vi "TypeToVariantForContextHelp.vi"(11 "Type":refnum<class "Type.lvclass">) -> (3 "Variant":variant)   [LabVIEW 2021]
uses:
  <vilib>/imath/engines/lvmath2/MathScriptCompiler/Type.llb/Type.lvclass
  <vilib>/imath/engines/lvmath2/MathScriptCompiler/Type/Matrix.llb/Matrix.lvclass
  C:/builds/2021/dev/dist/vi.lib/imath/engines/lvmath2/MathScriptCompiler/Type/NDArray.llb/NDArray.lvclass
  C:/builds/2021/dev/dist/vi.lib/imath/engines/lvmath2/MathScriptCompiler/Type.llb/Type.lvclass
  <vilib>/imath/engines/lvmath2/MathScriptCompiler/Type/BaseEltType.llb/BaseEltType.lvclass
  <vilib>/imath/engines/lvmath2/MathScriptCompiler/Type/PlugInEltType.llb/PlugInEltType.lvclass
  <vilib>/Utility/VariantDataType/MemoryInfo.ctl
  <vilib>/Utility/VariantDataType/MemoryType.ctl
  <vilib>/imath/engines/lvmath2/MathScriptCompiler/Type/NDArray.llb/NDArray.lvclass
  <vilib>/imath/engines/lvmath2/MathScriptCompiler/Type/StructEltType.llb/StructEltType.lvclass
  <vilib>/Utility/VariantDataType/VariantType.lvlib
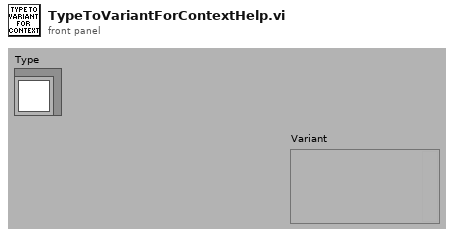
[diagram p1: front panel]
types:
  T1 = typedef "VariantType.lvlib/MemoryInfo.ctl" = cluster{"Type":T2, "Size":u32}
  T2 = typedef "VariantType.lvlib/MemoryType.ctl" = enum16{"Variable", "Fixed", "Bounded"}
  T3 = typedef "MathScriptTypes.lvlib/Matrix.lvclass/Shape.ctl" = enum16{"Scalar", "Row Vector", "Column Vector", "Matrix"}
  T4 = typedef "MathScriptTypes.lvlib/StructEltType.lvclass/StructField.ctl" = cluster{"Name":string, "Data Type":refnum<class "Type.lvclass">}
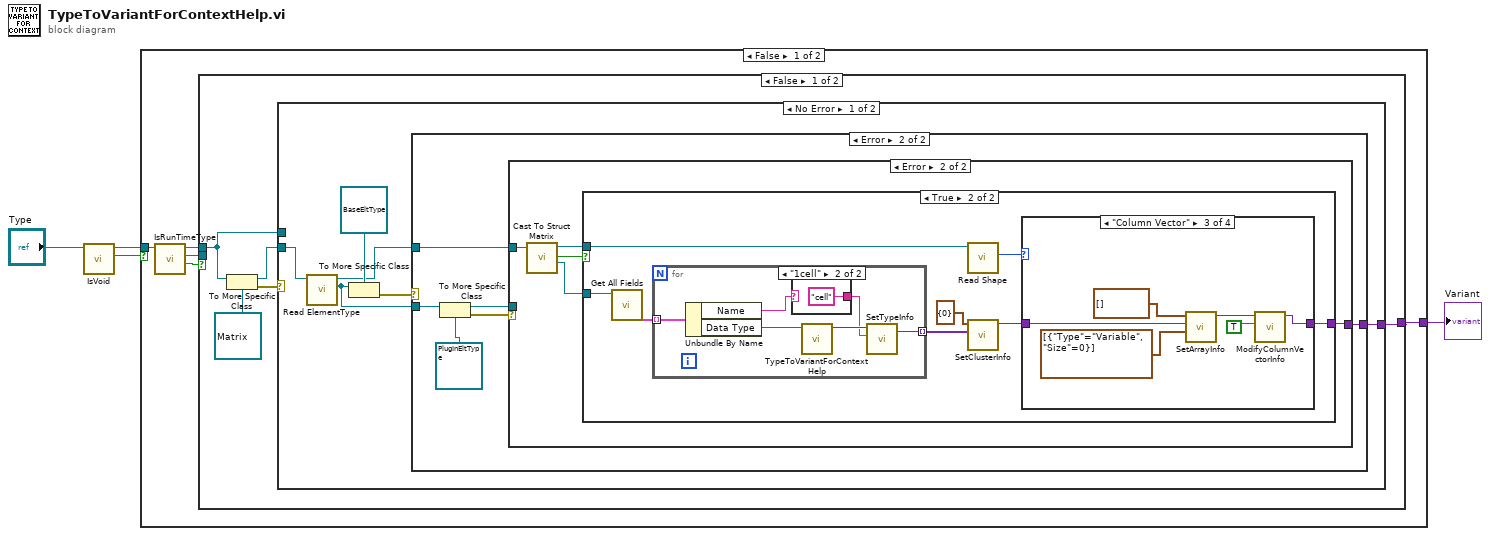
[diagram p0: block diagram]
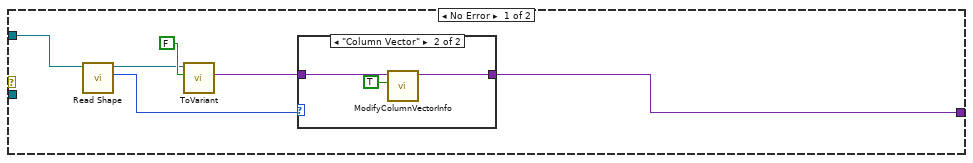
[diagram p2: hidden frame]
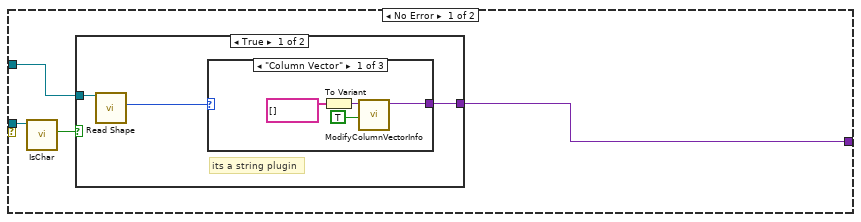
[diagram p4: hidden frame]
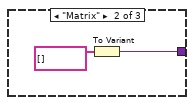
[diagram p5: hidden frame]
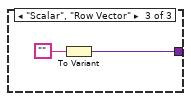
[diagram p6: hidden frame]
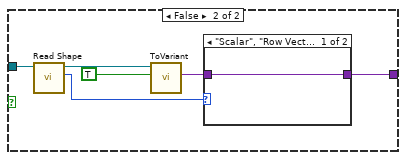
[diagram p7: hidden frame]
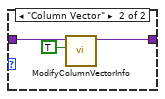
[diagram p8: hidden frame]
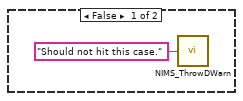
[diagram p9: hidden frame]
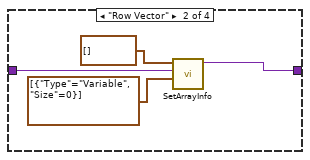
[diagram p11: hidden frame]
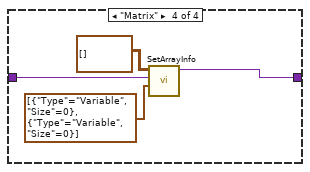
[diagram p12: hidden frame]
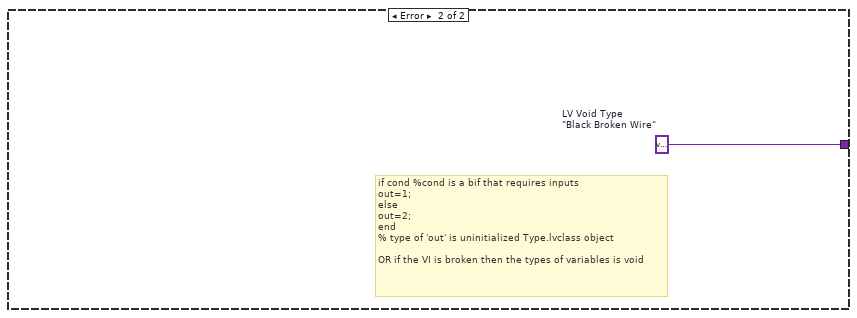
[diagram p14: hidden frame]
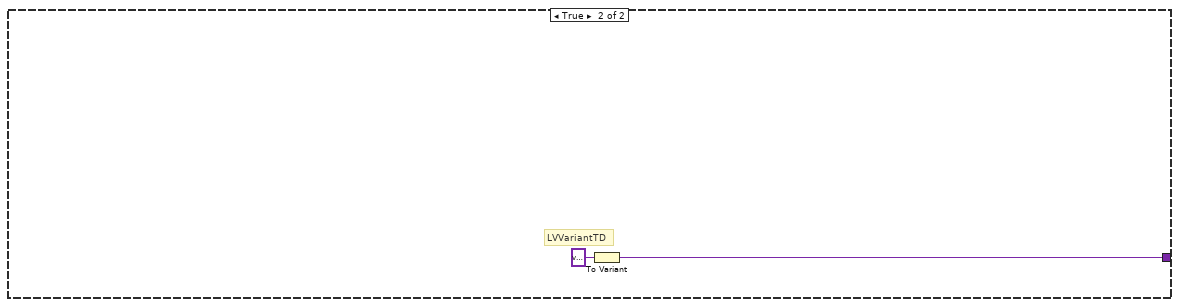
[diagram p15: hidden frame]
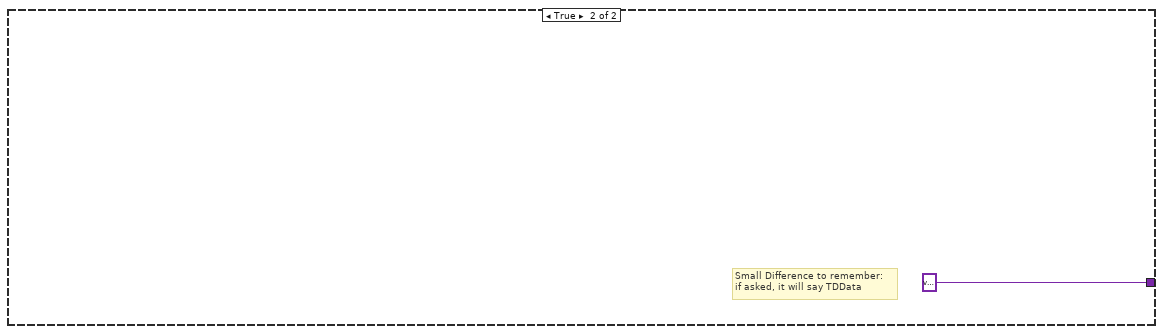
[diagram p16: hidden frame]
diagram:
  n1 = call-dynamic "IsVoid.vi"("Type in"="Type") -> ("IsVoid"=w1:bool, "Type out"=w2:refnum<class "Type.lvclass">)  [unwired: 9 in]
  n2 = case shown="False" w1 {
    tunnel: [w6 variant ("Variant")] -> w4
    tunnel: w2 -> [w5 _]
    frame False {
      n3 = call-dynamic "IsRunTimeType.vi"("Type"=w5) -> ("IsRunTimeType?"=w7:bool, "RunTimeType out"=w9:refnum<class "RuntimeType.lvclass">, "Type (dup)"=w8:refnum<class "Type.lvclass">)  [unwired: 8 out]
      n4 = case shown="False" w7 {
        tunnel: w9 -> [_ _]
        tunnel: w8 -> [w10 _]
        tunnel: [w11 w100] -> w6
        frame False {
          n5 = To More Specific Class(target class=refnum<class "Matrix.lvclass"> refnum ("Matrix out"), reference=w10) -> (specific class reference=w12:refnum<class "Matrix.lvclass">, error out=w13:errorcluster)  [unwired: 1 in]
          n6 = case shown="No Error" w13 {
            tunnel: w12 -> [w19 _]
            tunnel: [w15 w99] -> w11
            tunnel: w10 -> [_ _]
            frame No Error {
              n7 = call <vilib>:"Read ElementType.vi"("NDArray.lvclass in"=w19) -> ("ElementType"=w16:refnum<class "ElementType.lvclass">, "NDArray.lvclass out"=w17:refnum<class "Matrix.lvclass">)  [unwired: 9 out]
              n8 = To More Specific Class(target class=refnum<class "BaseEltType.lvclass"> refnum ("BaseEltType.lvclass in"), reference=w16) -> (error out=w18:errorcluster)  [unwired: 1 in, 1 out]
              n9 = case shown="Error" w18 {
                tunnel: w17 -> [w25 w32]
                tunnel: [w21 w31] -> w15
                tunnel: w16 -> [_ w35]
                frame No Error {
                  n10 = call <vilib>:"Read Shape.vi"("Matrix.lvclass in"=w25) -> ("Shape"=w23:T3, "Matrix.lvclass out"=w24:refnum<class "Matrix.lvclass">)  [unwired: 9 in]
                  n11 = call-dynamic "ToVariant.vi"("Set ColVector on TDR? (F)"=FALSE ("Ignore CondDefined?"), "Matrix in"=w24) -> ("Variant"=w22:variant)  [unwired: 2 in, 7 out]
                  n12 = case shown="\"Column Vector\"" w23 {
                    tunnel: w22 -> [w27 w28]
                    tunnel: [w27 w30] -> w21
                    frame "Scalar", "Row Vector", "Matrix" {
                    }
                    frame "Column Vector" {
                      n13 = call <vilib>:"ModifyColumnVectorInfo.vi"("isColumnVector"=TRUE, "Variant"=w28) -> ("Variant out"=w30:variant)  [unwired: 8 in, 1 out]
                    }
                  }
                }
                frame Error {
                  n14 = To More Specific Class(target class=refnum<class "PlugInEltType.lvclass"> refnum, reference=w35) -> (specific class reference=w33:refnum<class "PlugInEltType.lvclass">, error out=w34:errorcluster)  [unwired: 1 in]
                  n15 = case shown="Error" w34 {
                    tunnel: w33 -> [w38 _]
                    tunnel: w32 -> [w40 w66]
                    tunnel: [w39 w62] -> w31
                    frame No Error {
                      n16 = call-dynamic "IsChar.vi"("PlugInEltType in"=w38) -> ("Is Char?"=w37:bool)  [unwired: 9 in, 1 out]
                      n17 = case shown="True" w37 {
                        tunnel: w40 -> [w43 w57]
                        tunnel: [w41 w52] -> w39
                        frame True {
                          # "its a string plugin"
                          n18 = call <vilib>:"Read Shape.vi"("Matrix.lvclass in"=w43) -> ("Shape"=w42:T3)  [unwired: 9 in, 1 out]
                          n19 = case shown="\"Column Vector\"" w42 {
                            tunnel: [w47 w48 w50] -> w41
                            frame "Column Vector" {
                              n20 = To Variant(anything=string[] []) -> (Variant=w45:variant)
                              n21 = call <vilib>:"ModifyColumnVectorInfo.vi"("isColumnVector"=TRUE, "Variant"=w45) -> ("Variant out"=w47:variant)  [unwired: 8 in, 1 out]
                            }
                            frame "Matrix" {
                              n22 = To Variant(anything=string[] []) -> (Variant=w48:variant)
                            }
                            frame "Scalar", "Row Vector" {
                              n23 = To Variant(anything="") -> (Variant=w50:variant)
                            }
                          }
                        }
                        frame False {
                          n24 = call <vilib>:"Read Shape.vi"("Matrix.lvclass in"=w57) -> ("Shape"=w56:T3, "Matrix.lvclass out"=w55:refnum<class "Matrix.lvclass">)  [unwired: 9 in]
                          n25 = call-dynamic "ToVariant.vi"("Set ColVector on TDR? (F)"=TRUE ("Ignore CondDefined?"), "Matrix in"=w55) -> ("Variant"=w53:variant)  [unwired: 7 in, 2 out]
                          n26 = case shown="\"Scalar\", \"Row Vector\", \"Matrix\"" w56 {
                            tunnel: w53 -> [w58 w61]
                            tunnel: [w58 w60] -> w52
                            frame "Scalar", "Row Vector", "Matrix" {
                            }
                            frame "Column Vector" {
                              n27 = call <vilib>:"ModifyColumnVectorInfo.vi"("isColumnVector"=TRUE, "Variant"=w61) -> ("Variant out"=w60:variant)  [unwired: 8 in, 1 out]
                            }
                          }
                        }
                      }
                    }
                    frame Error {
                      n28 = call <vilib>:"Cast To Struct Matrix.vi"("Type in"=w66) -> ("IsStructMatrix?"=w65:bool, "StructEltType out"=w64:refnum<class "StructEltType.lvclass">, "Type (dup)"=w63:refnum<class "Matrix.lvclass">)  [unwired: 7 in, 1 out]
                      n29 = case shown="True" w65 {
                        tunnel: w64 -> [_ w75]
                        tunnel: w63 -> [_ w73]
                        tunnel: [_ w71] -> w62
                        frame False {
                          n30 = call <vilib>:"NIMS_ThrowDWarn.vi"("DWarn"="Should not hit this case.") -> ()  [unwired: 1 in]
                        }
                        frame True {
                          n31 = call <vilib>:"Get All Fields.vi"("StructEltType in"=w75) -> ("Fields"=w74:T4[])  [unwired: 8 in, 2 out]
                          n32 = for {
                            tunnel: w74 -> [w96] mode=indexing
                            tunnel: [w93] -> w69 mode=indexing
                            n33 = Unbundle By Name(w96) -> ("Name"=w92:string, "Data Type"=w95:refnum<class "Type.lvclass">)
                            n34 = case shown="\"1cell\"" w92 {
                              selector: w92 -> [w97 _]
                              tunnel: [w97 "cell"] -> w91
                              frame "False", Default {
                              }
                              frame "1cell" {
                              }
                            }
                            n35 = call <vilib>:"TypeToVariantForContextHelp.vi"("Type"=w95) -> ("Variant"=w94:variant)  [unwired: 10 in]
                            n36 = call <vilib>:"SetTypeInfo.vi"("Name"=w91, "Variant"=w94) -> ("Variant Out"=w93:variant)  [unwired: 8 in, 1 out]
                          }
                          n37 = call <vilib>:"Read Shape.vi"("Matrix.lvclass in"=w73) -> ("Shape"=w72:T3)  [unwired: 9 in, 1 out]
                          n38 = call <vilib>:"SetClusterInfo.vi"("Cluster Elements"=w69, "Variant"=cluster{i32} {0}) -> ("Variant Out"=w68:variant)  [unwired: 8 in, 1 out]
                          n39 = case shown="\"Column Vector\"" w72 {
                            tunnel: [w76 w78 w81 w88] -> w71
                            tunnel: w68 -> [w76 w80 w86 w89]
                            frame "Scalar" {
                            }
                            frame "Row Vector" {
                              n40 = call <vilib>:"SetArrayInfo.vi"("Array Lengths"=T1[] [{"Type"=enum."Variable", "Size"=0}], "Array Element"=w80, "Variant"=cluster{i32}[] []) -> ("Variant Out"=w78:variant)  [unwired: 7 in, 1 out]
                            }
                            frame "Column Vector" {
                              n41 = call <vilib>:"SetArrayInfo.vi"("Array Lengths"=T1[] [{"Type"=enum."Variable", "Size"=0}], "Array Element"=w86, "Variant"=cluster{i32}[] []) -> ("Variant Out"=w82:variant)  [unwired: 7 in, 1 out]
                              n42 = call <vilib>:"ModifyColumnVectorInfo.vi"("isColumnVector"=TRUE, "Variant"=w82) -> ("Variant out"=w81:variant)  [unwired: 8 in, 1 out]
                            }
                            frame "Matrix" {
                              n43 = call <vilib>:"SetArrayInfo.vi"("Array Lengths"=T1[] [{"Type"=enum."Variable", "Size"=0}, {"Type"=enum."Variable", "Size"=0}], "Array Element"=w89, "Variant"=cluster{i32}[][] []) -> ("Variant Out"=w88:variant)  [unwired: 7 in, 1 out]
                            }
                          }
                        }
                      }
                    }
                  }
                }
              }
            }
            frame Error {
              w99 = variant  # LV Void Type "Black Broken Wire"
              # "if cond %cond is a bif that requires inputs\nout=1;\nelse\nout=2;\nend\n% type of 'out' is uninitialized Type.lvclass object\n\nOR if the VI is broken then the types of variables is void"
            }
          }
        }
        frame True {
          # "LVVariantTD"
          n44 = To Variant(anything=variant ("Variant")) -> (Variant=w100:variant)
        }
      }
    }
    frame True {
      # "Small Difference to remember:\nif asked, it will say TDData"
    }
  }
  "Variant" <- w4
